vi "Calculate Due Dates.vi"(8 "error in (no error)":errorcluster, 11 "OSSP_Problem in":refnum<class "OSSP_Problem.lvclass">) -> (0 "error out":errorcluster, 3 "OSSP_Problem out":refnum<class "OSSP_Problem.lvclass">)   [LabVIEW 2013, in "OSSP_Problem.lvclass"]
uses:
  OSSP_Problem.lvclass
  OSSP_Problem.lvclass/OSSP_Problem.ctl
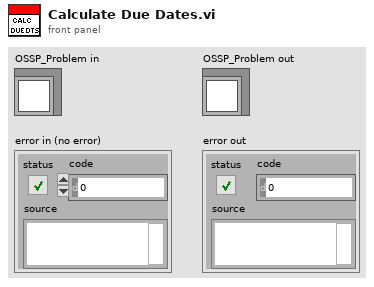
[diagram p1: front panel]
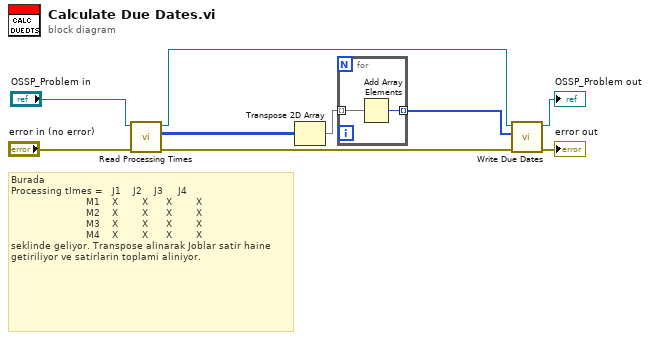
[diagram p0: block diagram]
diagram:
  # "Burada \nProcessing tImes =   J1    J2    J3     J4   \n                         M1    X        X      X        X\n                         M2    X        X      X        X\n                         M3    X        X      X        X\n                         M4    X        X      X        X\nseklinde geliyor. Transpose alinarak Joblar satir haine getiriliyor ve satirlarin toplami aliniyor."
  n1 = call "Read Processing Times.vi"("error in (no error)"="error in (no error)", "OSSP_Problem in"="OSSP_Problem in") -> ("error out"=w5:errorcluster, "Processing Times"=w2:u16[][], "OSSP_Problem out"=w4:refnum<class "OSSP_Problem.lvclass">)  [unwired: 7 in]
  n2 = Transpose 2D Array(2D array=w2) -> (transposed array=w3:u16[][])
  n3 = for {
    tunnel: w3 -> [w11] mode=indexing
    tunnel: [w10] -> w1 mode=indexing
    n4 = Add Array Elements(numeric array=w11) -> (sum=w10:u16)
  }
  n5 = call "Write Due Dates.vi"("error in (no error)"=w5, "Due Dates"=w1, "OSSP_Problem in"=w4) -> ("error out"=→"error out":errorcluster, "OSSP_Problem out"=→"OSSP_Problem out":refnum<class "OSSP_Problem.lvclass">)  [unwired: 7 in]
